vi "setUp.vi"(8 "error in (no error)":errorcluster, 11 "reference in":refnum<class "Read File Tests.lvclass">) -> (0 "error out":errorcluster, 3 "reference out":refnum<class "Read File Tests.lvclass">)   [LabVIEW 2017, in "Read File Tests.lvclass"]
doc: "setUp runs prior to the test method during test execution. Use this method to initialize any object data required by your tests."
uses:
  Read File Tests.lvclass
  Read File Tests.lvclass/Read File Tests.ctl
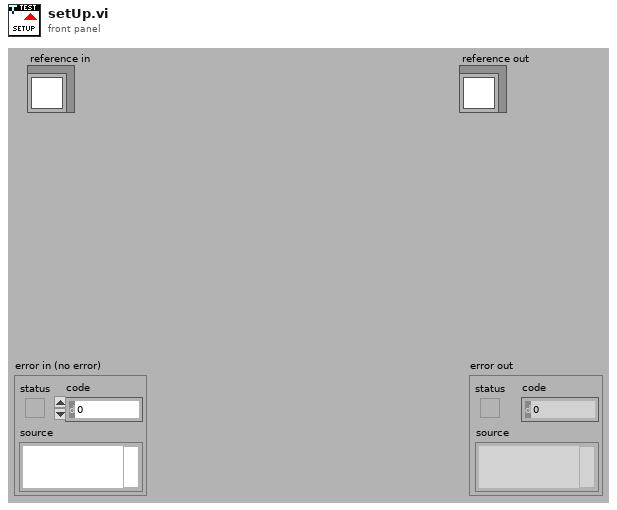
[diagram p1: front panel]
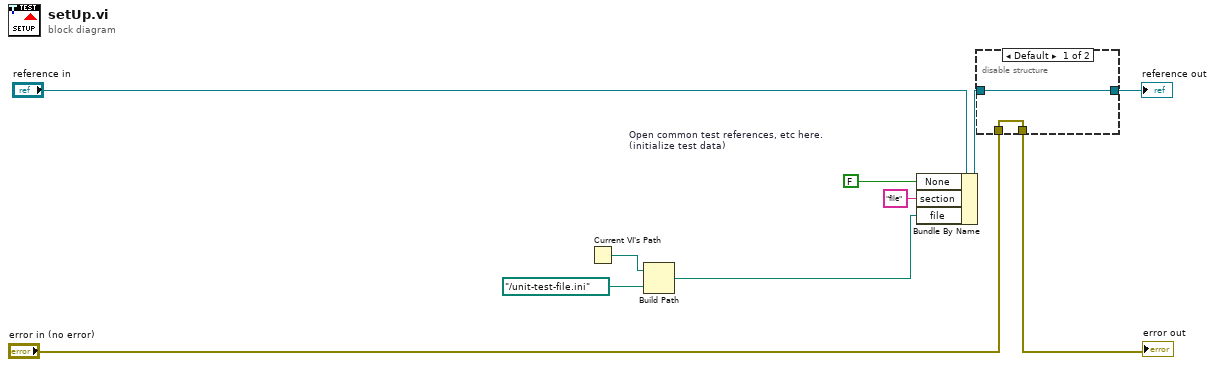
[diagram p0: block diagram]
diagram:
  w6 = FALSE  # Open common test references, etc here. (initialize test data)
  n1 = Current VI's Path() -> (path=w4:path)
  n2 = Build Path(base path=w4, name or relative path=path "../unit-test-file.ini") -> (appended path=w1:path)
  n3 = Bundle By Name(cluster="reference in", "None"=w6, "section"="file", "file"=w1) -> (w7:refnum<class "Read File Tests.lvclass">)
  n4 = disable-structure shown="Default" {
    disable-tunnel: "error in (no error)" -> [w11 w13]
    disable-tunnel: [w11 w13] -> w10
    disable-tunnel: [w12 w14] -> w8
    disable-tunnel: w7 -> [w12 w14]
    frame condition #0 (active) {
    }
    frame condition #1 {
    }
  }
  "error out" <- w10
  "reference out" <- w8
